vi "Create and Format Image Structure.vi"(4 "Max Height (50 pixels)":i16=50, 6 "Max Width (500 pixels)":i16=500, 7 "Name Addition":string, 8 "Error in":errorcluster caption="Error in (no error)", 9 "Image Data":T1, 10 "Name":string, 11 "VIDoc Printer - Confluence In":refnum<class "VIDoc Printer - Confluence.lvclass">) -> (0 "Error out":errorcluster, 1 "Image Created?":bool, 2 "Image Structure Text":string, 3 "VIDoc Printer - Confluence Out":refnum<class "VIDoc Printer - Confluence.lvclass">)   [LabVIEW 2023, in "VIDoc Printer - Confluence.lvlib" / "VIDoc Printer - Confluence.lvclass"]
uses:
  VIDoc Printer - Confluence.lvclass
  <vilib>/picture/picture.llb/imagedata.ctl
  VIDoc Printer - Confluence.lvclass/VIDoc Printer - Confluence.ctl
  Accessors/Get Temporary Image Directory+.vi
  <vilib>/Utility/libraryn.llb/Create Directory Recursive.vi
  Printer/VIDoc Printer.lvclass
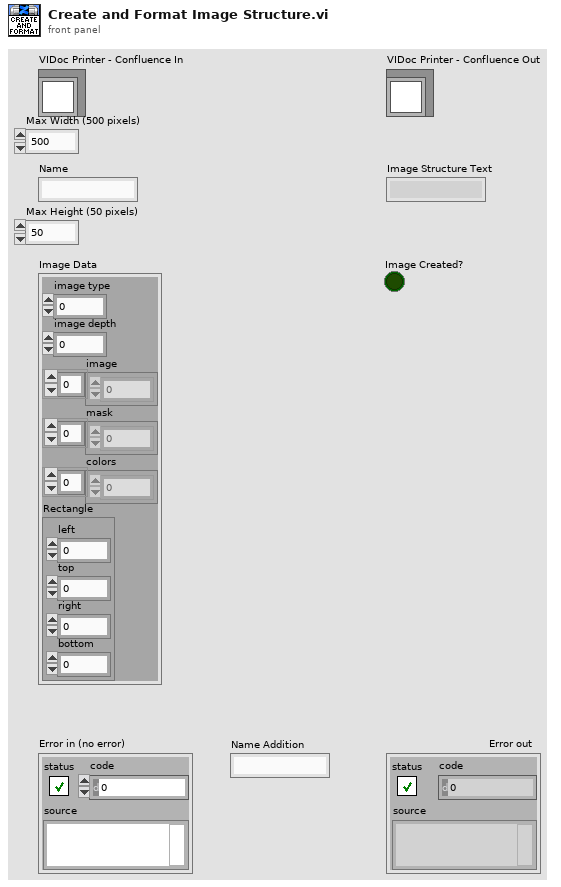
[diagram p1: front panel]
types:
  T1 = typedef "imagedata.ctl" = cluster{"image type":i32, "image depth":i32, "image":u8[], "mask":u8[], "colors":u32[], "Rectangle":cluster{"left":i16, "top":i16, "right":i16, "bottom":i16}}
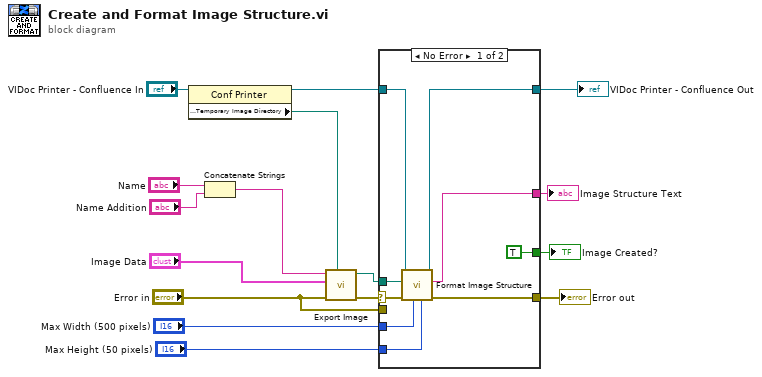
[diagram p0: block diagram]
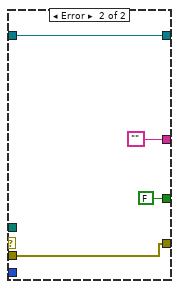
[diagram p2: hidden frame]
diagram:
  n1 = property class="Conf Printer"(reference="VIDoc Printer - Confluence In") -> (reference out=w4:refnum<class "VIDoc Printer - Confluence.lvclass">, "Properties:Temporary Image Directory"=w3:path)  [unwired: 1 in, 1 out]
  n2 = Concatenate Strings("Name", "Name Addition") -> (w14:string)
  n3 = call "Export Image.vi"("Temporary Image Directory"=w3, "Error in"="Error in", "Image Data"="Image Data", "Name"=w14) -> ("Error out"=w16:errorcluster, "Image Path"=w15:path)  [unwired: 6 in]
  n4 = case shown="No Error" w16 {
    selector: w16 -> [w25 _]
    tunnel: w15 -> [w24 _]
    tunnel: [w23 w29] -> w7
    tunnel: [w22 w27] -> w8
    tunnel: w4 -> [w21 w27]
    tunnel: [w20 ""] -> w6
    tunnel: [TRUE ("File Change Info Available?") FALSE ("File Change Info Available?")] -> w5
    tunnel: "Error in" -> [_ w29]
    tunnel: "Max Width (500 pixels)" -> [w18 _]
    tunnel: "Max Height (50 pixels)" -> [w17 _]
    frame No Error {
      n5 = call "Format Image Structure.vi"("Max Height (50 pixels)"=w17, "Max Width (500 pixels)"=w18, "error in (no error)"=w25, "Image"=w24, "VIDoc Printer - Confluence In"=w21) -> ("error out"=w23:errorcluster, "Image Structure Text"=w20:string, "VIDoc Printer - Confluence Out"=w22:refnum<class "VIDoc Printer - Confluence.lvclass">)  [unwired: 4 in]
    }
    frame Error {
    }
  }
  "Error out" <- w7
  "VIDoc Printer - Confluence Out" <- w8
  "Image Structure Text" <- w6
  "Image Created?" <- w5
